vi "XCP and CCP - Curve Table Control.vi"() -> ()   [LabVIEW 2011]
doc: "Sample numeric display item."
uses:
  <vilib>/NI Veristand/Display Template Support/Display Template Support.llb/cluster_Screen Item Settings.ctl
  <vilib>/NI Veristand/Display Template Support/Display Template Support.llb/cluster_Graph Scale Settings.ctl
  <vilib>/NI Veristand/Display Template Support/Display Template Support.llb/cluster_Graph Plot Settings.ctl
  NationalInstruments.VeriStand.SystemStorage
  Tables/XCPCCP TBL1D.xctl
  Controls/Control Links.ctl
  Controls/ECUMC Item.ctl
  <vilib>/NI Veristand/Display Template Support/Display Template Support.llb/enum_Display Template Handler Minimal To Widget Msg.ctl
  <vilib>/NI Veristand/Display Template Support/Display Template Support.llb/enum_Display Template Handler Minimal To Workspace.ctl
  Controls/All Link Data.ctl
  Controls/LinkData.ctl
  <vilib>/ECUMC/NIVS/Support Files.llb/Item Properties.ctl
  <vilib>/ECUMC/NIVS/Support Files.llb/Address Property.ctl
  <vilib>/ECUMC/NIVS/Support Files.llb/Extension Property.ctl
  <vilib>/ECUMC/NIVS/Support Files.llb/Data Type Property.ctl
  <vilib>/ECUMC/NIVS/Support Files.llb/Byte Order Property.ctl
  <vilib>/ECUMC/NIVS/Support Files.llb/Maximum Property.ctl
  <vilib>/ECUMC/NIVS/Support Files.llb/Minimum Property.ctl
  <vilib>/ECUMC/NIVS/Support Files.llb/Read Only Property.ctl
  <vilib>/ECUMC/NIVS/Support Files.llb/Unit Property.ctl
  <vilib>/ECUMC/NIVS/Support Files.llb/Comment Property.ctl
  <vilib>/ECUMC/NIVS/Support Files.llb/X Dimension Property.ctl
  <vilib>/ECUMC/NIVS/Support Files.llb/Y Dimension Property.ctl
  <vilib>/ECUMC/NIVS/Support Files.llb/Is Virtual Property.ctl
  Tables/Limits TBL1D.ctl
  <vilib>/ECUMC/NIVS/Support Files.llb/Item Type.ctl
  SubVIs/Get Conn Status Chan Path.vi
  SubVIs/Check Link for Char or Meas.vi
  <vilib>/NI Veristand/Display Template Support/Display Template Support.llb/sub_Display Template Handler Custom.vi
  <vilib>/ECUMC/NIVS/Set Char Data.vi
  <vilib>/ECUMC/NIVS/Support Files.llb/Set Char Data (1d, TCP).vi
  <vilib>/NI Veristand/Execution/Workspace/NI VeriStand - Set Channel Value.vi
  <vilib>/NI Veristand/Execution/Workspace/NI VeriStand - Set Multiple Channel Values.vi
  <vilib>/NI Veristand/Execution/Workspace/NI VeriStand - Get Channel Value.vi
  <vilib>/NI Veristand/Execution/Workspace/NI VeriStand - Get Multiple Channel Values.vi
  <vilib>/NI Veristand/Execution/Workspace/NI VeriStand - Get System State.vi
  <vilib>/ECUMC/NIVS/Support Files.llb/Get Single Char Properties (TCP).vi
  <vilib>/ECUMC/NIVS/Get Char Data.vi
  <vilib>/ECUMC/NIVS/Support Files.llb/Get Single Char Data (TCP).vi
  <vilib>/ECUMC/NIVS/Get Meas Data.vi
  <vilib>/ECUMC/NIVS/Support Files.llb/Get Single Meas Data (TCP).vi
  <vilib>/NI Veristand/Execution/Workspace/NI VeriStand - Get Single Channel Value.vi
  <vilib>/NI Veristand/Execution/Workspace/NI_VS Workspace ExecutionAPI.lvlib
  <vilib>/ECUMC/NIVS/XCPCCP Add-On Execution API.lvlib
  <vilib>/ECUMC/NIVS/Support Files.llb/XCP and CCP Master Custom Device.lvlib
panel:
  in  "Links":T1
  out "Selected Parameter":string
  in  "TBL1D":cluster{"X":sgl[], "Y":sgl[]}(xcontrol)
  in  "NIVS.System Definition Root":refnum<k24>
  in  "Item.Data":T3
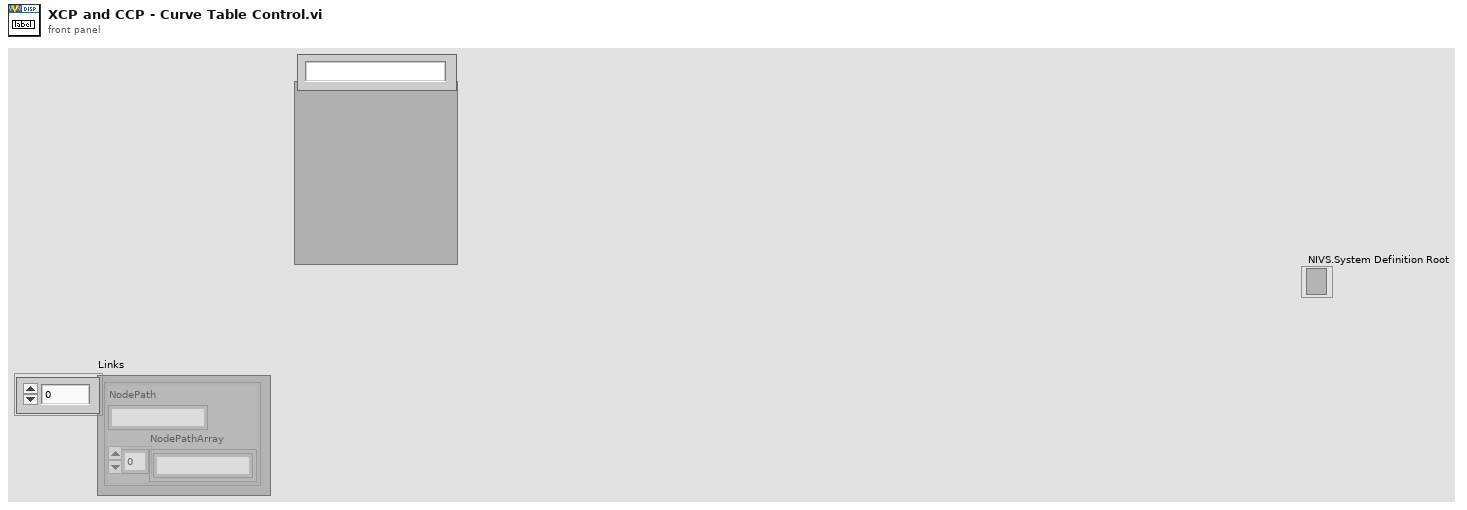
[diagram p1: front panel]
types:
  T1 = typedef "Control Links.ctl" = T2[]
  T2 = typedef "ECUMC Item.ctl" = cluster{"NodePath":string, "NodePathArray":string[]}
  T3 = typedef "cluster_Screen Item Settings.ctl" = cluster{"Template VI":string, "Position X":i32, "Position Y":i32, "Custom":string, "Show Title Bar":bool, "ID":i32, "Always On Top":bool, "Allow Resize":bool, "Allow Minimize":bool, "Allow Close":bool, "Size to Screen":bool, "Screen.ID":i32, "State":enum16{"Normal", "New"}, "Title":string, "Window Bounds":cluster{"[0]":i16, "[1]":i16, "[2]":i16, "[3]":i16}, "Channel Ref":u64, "Unit":string, "Default Units?":bool, "Flash Limit?":bool, "Color 1":u32, "Color 2":u32, "Color 3":u32, "Color 4":u32, "Bck Color":u32, "Fore Color":u32, "Limit 1":dbl, "Limit 2":dbl, "Limit 3":dbl, "Limit 4":dbl, "Limit Mode 1":i32, "Limit Mode 2":i32, "Limit Mode 3":i32, "Limit Mode 4":i32, "Scale Precision":i32, "Scale Min":dbl, "Scale Max":dbl, "Format":i32, "Precision":i32, "Background Type":i32, "IDs":i32[], "Units":string[], "Labels":string[], "Scale Factor":dbl, "Scale Offset":dbl, "YScale Index":u32[], "XScale":T4, "YScales":T4[], "Plots":T5[], "Update Period":dbl, "History Length":dbl, "My.Ref":refnum<vi>, "Is Control?":bool, "Channel Paths":string[], "Custom Data":variant}
  T4 = typedef "cluster_Graph Scale Settings.ctl" = cluster{"Format":u8, "Precision":u8, "Fit":u8, "Label":string, "Use Default Label":bool, "Label Visible":bool, "Min":dbl, "Max":dbl}
  T5 = typedef "cluster_Graph Plot Settings.ctl" = cluster{"Bar Style":u8, "Fill To":i16, "Fill/PtColor":u32, "Line Style":u8, "Line Width":u8, "Color":u32, "Interp":u8, "Point Style":u8}
  T6 = typedef "XCPCCP TBL1D.xctl/Limits TBL1D.ctl" = cluster{"Min X":sgl, "Max X":sgl, "MaxDiff X":sgl, "MaxGrad X":sgl, "Min Y":sgl, "Max Y":sgl, "MaxDiff Y":sgl}
  T7 = typedef "XCP and CCP Master Custom Device.lvlib/Item Properties.ctl" = cluster{"Common":cluster{"Address":T8, "Extension":T9, "Data Type":T10, "Byte Order":T11, "Maximum":T12, "Minimum":T13, "Read Only?":T14, "Unit":T15, "Comment":T16}, "Char Specific":cluster{"X Dimension":T17, "Y Dimension":T18, "char x axis":dbl[], "char y axis":dbl[], "char sizes":u32[]}, "Meas Specific":cluster{"Virtual?":T19}}
  T8 = typedef "XCP and CCP Master Custom Device.lvlib/Address Property.ctl" = u32
  T9 = typedef "XCP and CCP Master Custom Device.lvlib/Extension Property.ctl" = u8
  T10 = typedef "XCP and CCP Master Custom Device.lvlib/Data Type Property.ctl" = enum16{"UBYTE", "SBYTE", "UWORD", "SWORD", "ULONG", "SLONG", "FLOAT32_IEEE", "FLOAT64_IEEE"}
  T11 = typedef "XCP and CCP Master Custom Device.lvlib/Byte Order Property.ctl" = enum16{"Intel", "Motorola"}
  T12 = typedef "XCP and CCP Master Custom Device.lvlib/Maximum Property.ctl" = dbl
  T13 = typedef "XCP and CCP Master Custom Device.lvlib/Minimum Property.ctl" = dbl
  T14 = typedef "XCP and CCP Master Custom Device.lvlib/Read Only Property.ctl" = bool
  T15 = typedef "XCP and CCP Master Custom Device.lvlib/Unit Property.ctl" = string
  T16 = typedef "XCP and CCP Master Custom Device.lvlib/Comment Property.ctl" = string
  T17 = typedef "XCP and CCP Master Custom Device.lvlib/X Dimension Property.ctl" = u32
  T18 = typedef "XCP and CCP Master Custom Device.lvlib/Y Dimension Property.ctl" = u32
  T19 = typedef "XCP and CCP Master Custom Device.lvlib/Is Virtual Property.ctl" = bool
  T20 = typedef "All Link Data.ctl" = T21[]
  T21 = typedef "LinkData.ctl" = cluster{"Chns":string[], "InSys?":bool, "IP":string, "Port":u16}
  T22 = typedef "enum_Display Template Handler Minimal To Workspace.ctl" = cluster{"Operation":enum16{"SetCustomData", "DeleteItem"}, "Data":variant}
  T23 = typedef "enum_Display Template Handler Minimal To Widget Msg.ctl" = enum16{"Stop", "LaunchConfigDialog"}
  T24 = typedef "NI_VS Workspace ExecutionAPI.lvlib/WorkspaceAPI.ctl" = refnum<k24>
  T25 = typedef "NI_VS Workspace ExecutionAPI.lvlib/SystemStateEventRef.ctl" = cluster{"CustDatRef":refnum<user-event>, "EvtRef":refnum<k27>}
  T26 = typedef "NI_VS Workspace ExecutionAPI.lvlib/SystemStateRegEventRef.ctl" = refnum<event-registration>
  T27 = cluster{"Event Registration Refnum":refnum<event-registration>, "SystemChangeEventRef":T26}
  T28 = typedef "XCP and CCP Master Custom Device.lvlib/Item Type.ctl" = enum16{"Scalar Characteristic", "Curve Characteristic", "Field Characteristic", "Measurement"}
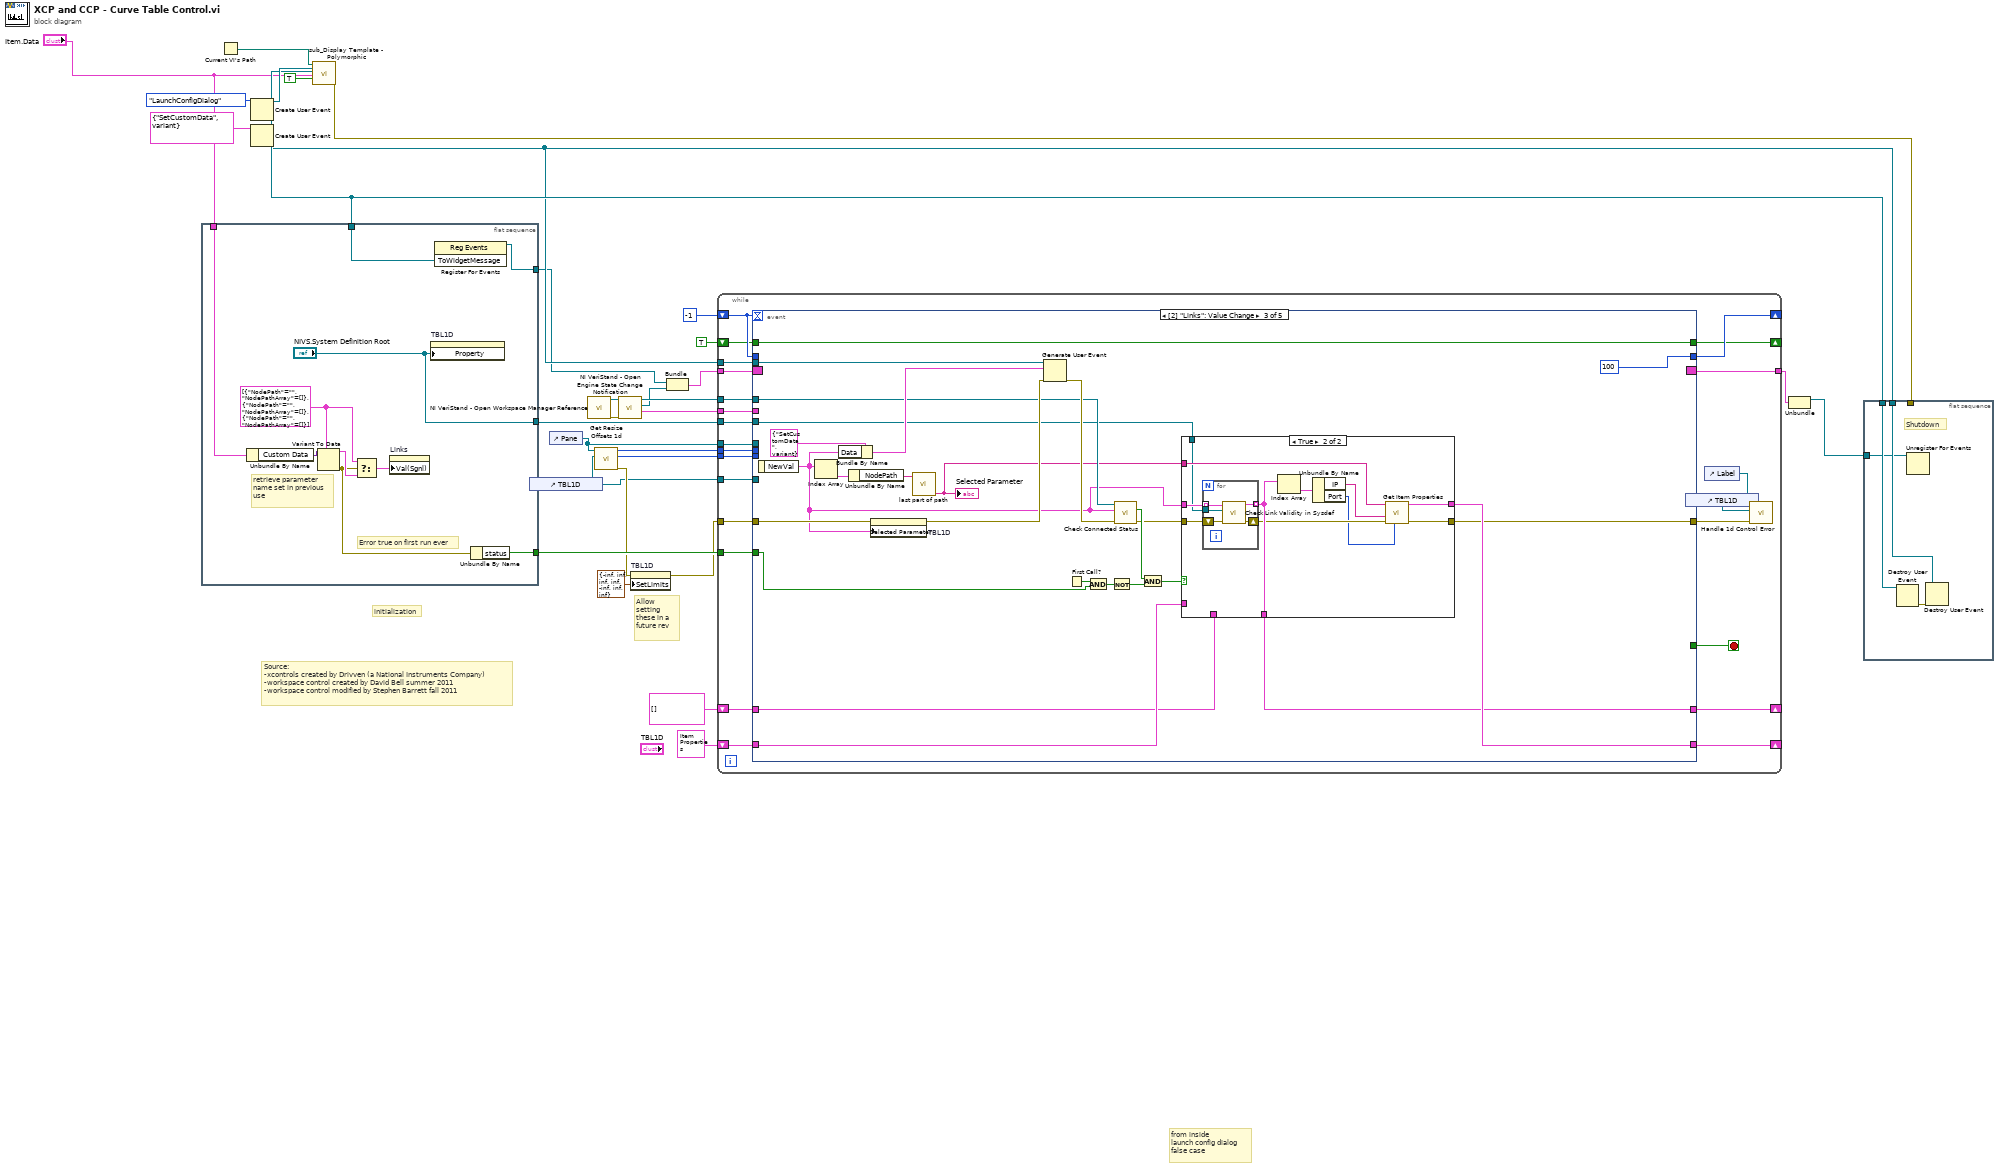
[diagram p0: block diagram]
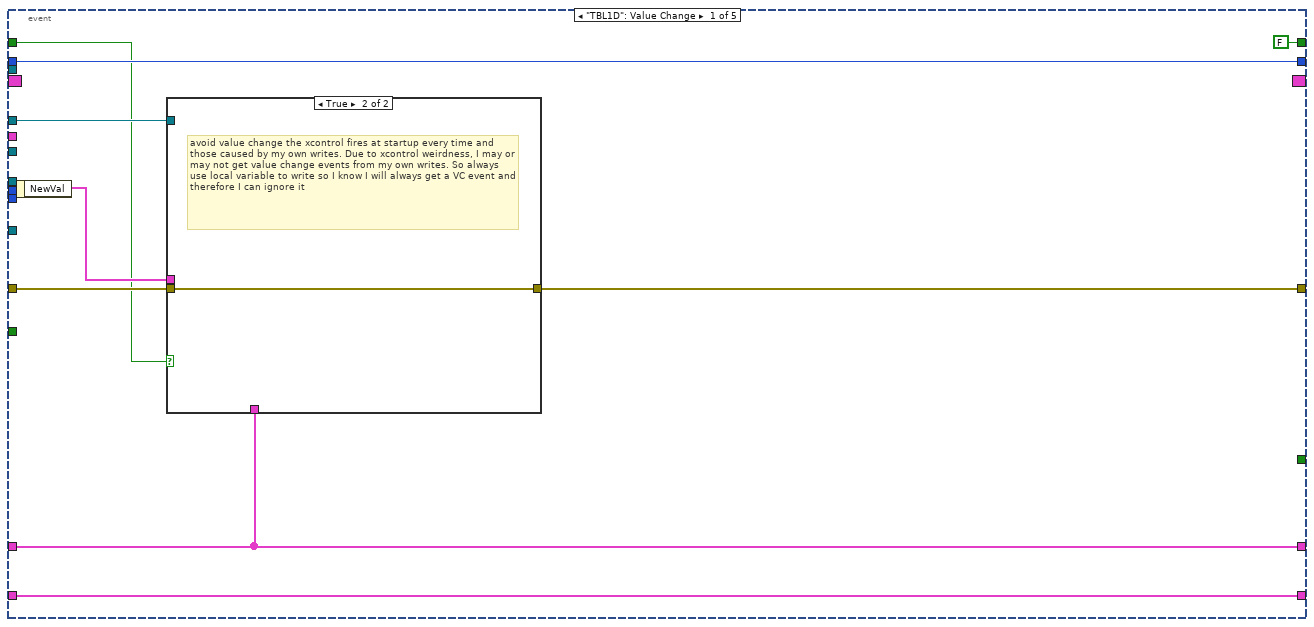
[diagram p2: hidden frame]
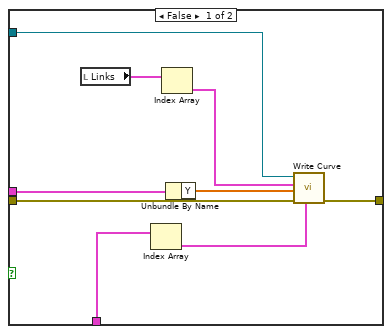
[diagram p3: hidden frame]
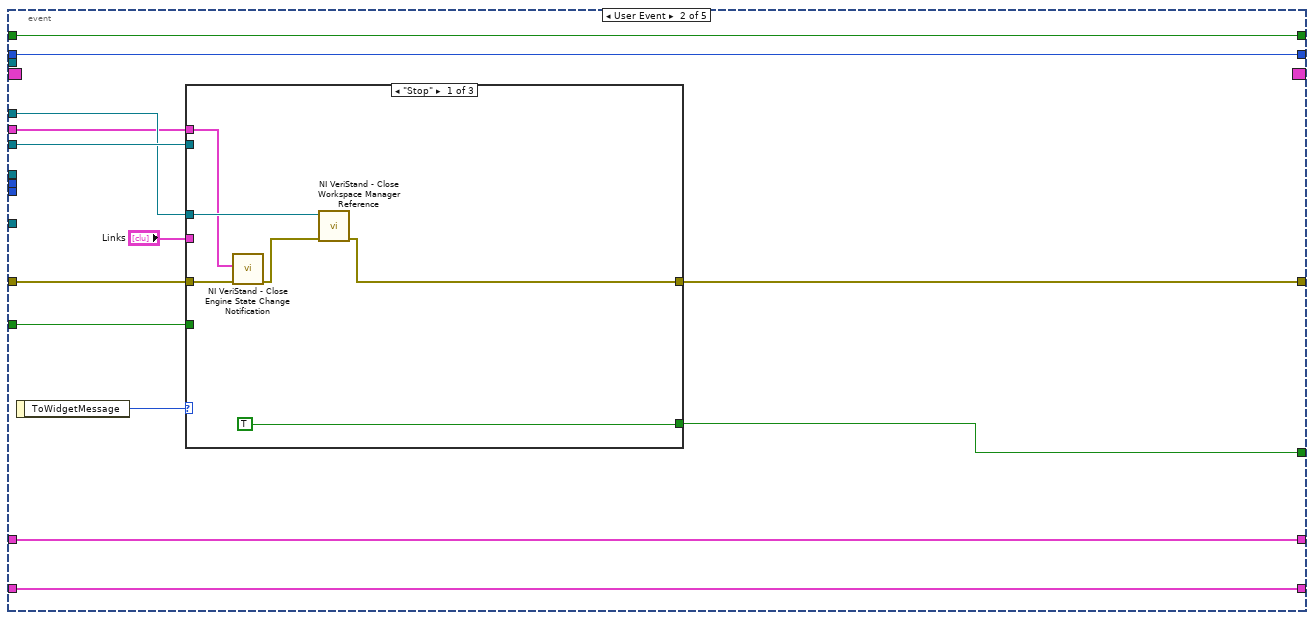
[diagram p4: hidden frame]
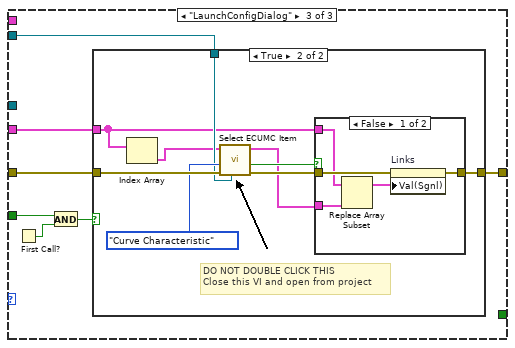
[diagram p6: hidden frame]
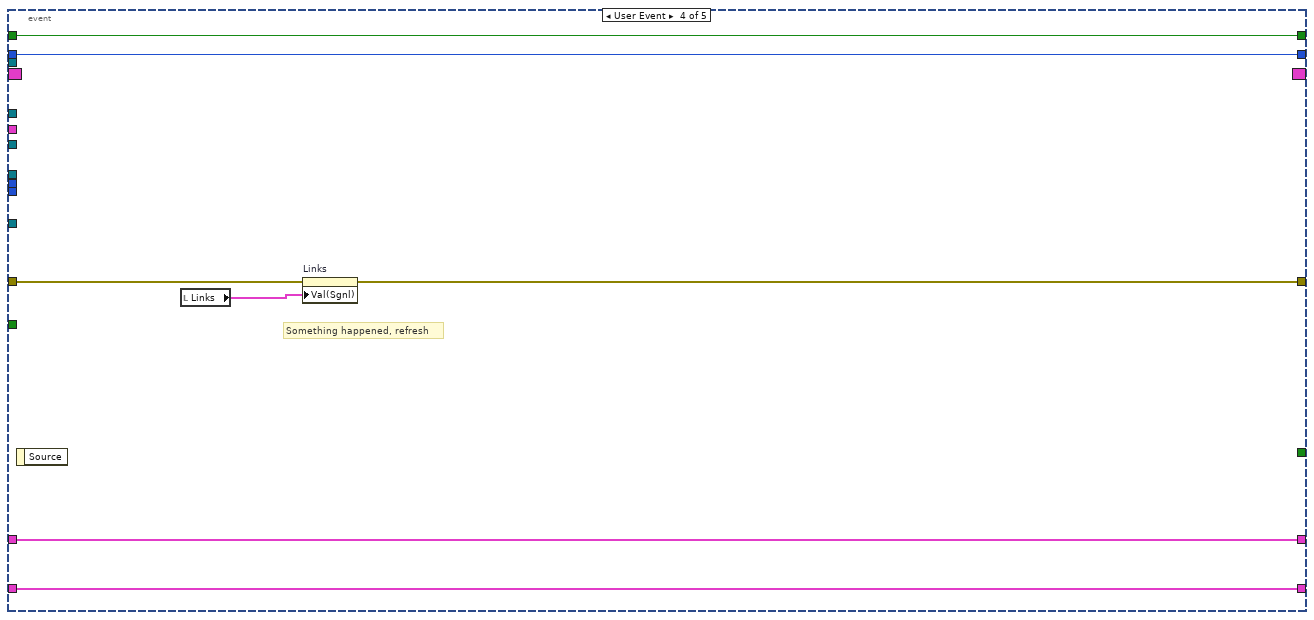
[diagram p10: hidden frame]
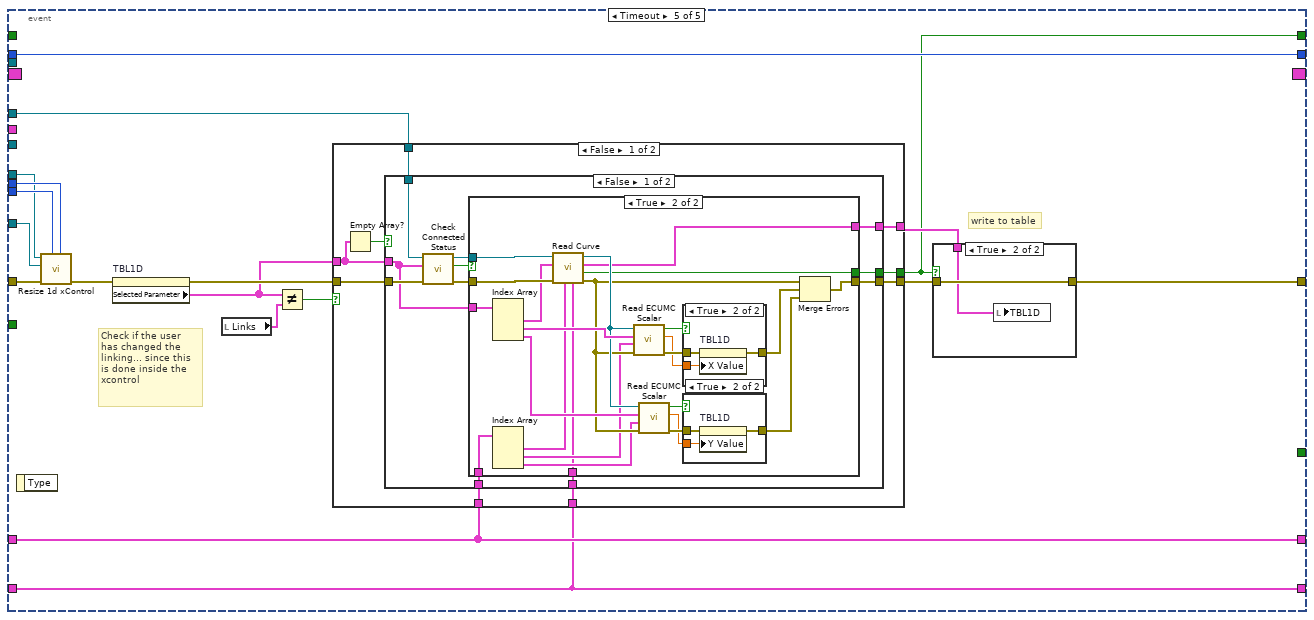
[diagram p11: hidden frame]
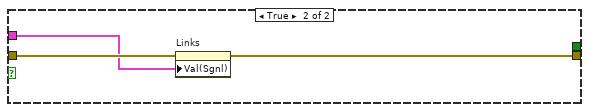
[diagram p17: hidden frame]
diagram:
  # "Source: \n-xcontrols created by Drivven (a National Instruments Company)\n-workspace control created by David Bell summer 2011\n-workspace control modified by Stephen Barrett fall 2011"
  # "Allow setting these in a future rev"
  # "initialization"
  # "from inside\nlaunch config dialog\nfalse case"
  n1 = flat-sequence {
    tunnel: [w40] -> w11
    tunnel: w28 -> [w39]
    tunnel: "Item.Data" -> [w37]
    tunnel: ["NIVS.System Definition Root"] -> w22
    tunnel: [w32] -> w21
    frame #0 {
      w31 = T1 [{"NodePath"="", "NodePathArray"=[]}, {"NodePath"="", "NodePathArray"=[]}, {"NodePath"="", "NodePathArray"=[]}] ("Links")
      # "Error true on first run ever"
      # "retrieve parameter\nname set in previous\nuse"
      n2 = Unbundle By Name(w37) -> ("Custom Data"=w38:variant)
      n3 = Variant To Data(type=w31, Variant=w38) -> (data=w34:T1, error out=w33:errorcluster)  [unwired: 1 in]
      n4 = Select(t=w31, s=w33, f=w34) -> (s? t:f=w35:T1)
      n5 = property on="Links" class="Arr (strict)"("Val(Sgnl)"=w35) -> ()  [unwired: 2 in, 2 out]
      n6 = property on="TBL1D" class="XCPCCP TBL1D (strict)"("Property"="NIVS.System Definition Root") -> ()  [unwired: 2 in, 2 out]
      n7 = register-events(w39) -> (reference out=w40:refnum<event-registration>)  [unwired: 2 in, 1 out]
      n8 = Unbundle By Name(w33) -> ("status"=w32:bool)
    }
  }
  n9 = Current VI's Path() -> (path=w26:path)
  n10 = Create User Event(user event datatype=enum_Display_Template_Handler_Minimal_To_Widget_Msg."LaunchConfigDialog" ("ToWidgetMessage")) -> (user event=w28:refnum<user-event>)  [unwired: 1 in, 1 out]
  n11 = Create User Event(user event datatype=T22 {"Operation"=enum."SetCustomData", "Data"=variant} ("Data")) -> (user event=w25:refnum<user-event>)  [unwired: 1 in, 1 out]
  n12 = call-poly <vilib>:"sub_Display Template - Polymorphic.vi"("Parent.Path"=w26, "ToWidgetEvent"=w28, "ToWorkspace"=w25, "Item.Data"="Item.Data", "Resizable"=TRUE) -> ("error out"=w30:errorcluster)  [unwired: 1 in, 13 out]
  n13 = control-ref of="TBL1D"() -> (w5:refnum<vi>)
  n14 = control-ref of="Pane"() -> (w16:refnum<vi>)
  n15 = call <vilib>:"NI VeriStand - Open Workspace Manager Reference.vi"() -> ("error out"=w13:errorcluster, "WorkspaceManager"=w12:T24)  [unwired: 10 in]
  n16 = call "Get Resize Offsets 1d.vi"("TBL1D Refnum"=w5, "Pane in"=w16) -> ("error out"=w19:errorcluster, "Width Offset"=w17:u32, "Height Offset"=w18:u32)  [unwired: 7 in]
  n17 = call <vilib>:"NI VeriStand - Open Engine State Change Notification.vi"("error in (no error)"=w13, "WorkspaceManager in"=w12) -> ("SystemStateRefs"=w7:T25, "SystemChangeEventRef"=w9:T26, "WorkspaceManager out"=w10:T24)  [unwired: 6 in, 1 out]
  n18 = property on="TBL1D" class="XCPCCP TBL1D (strict)"(error in=w19, "SetLimits"=T6 {"Min X"=-inf, "Max X"=inf, "MaxDiff X"=inf, "MaxGrad X"=inf, "Min Y"=-inf, "Max Y"=inf, "MaxDiff Y"=inf}) -> (error out=w20:errorcluster)  [unwired: 1 in, 1 out]
  n19 = Bundle("Event Registration Refnum"=w11, "SystemChangeEventRef"=w9) -> (w8:T27)  [unwired: 1 in]
  n20 = while {
    tunnel: w8 -> [w64]
    tunnel: [w63] -> w6
    tunnel: w25 -> [w62]
    tunnel: w20 -> [w60]
    tunnel: w10 -> [w61]
    tunnel: w22 -> [w59]
    tunnel: w21 -> [w58]
    tunnel: w18 -> [w57]
    tunnel: w17 -> [w56]
    tunnel: w16 -> [w55]
    tunnel: w5 -> [w54]
    shift-right: [w48] -> _
    shift-left: T20 [] ("All LinkData") -> [w46]
    shift-right: [w49] -> _
    shift-left: T7 {"Common"={"Address"=0, "Extension"=0, "Data Type"=enum."UBYTE", "Byte Order"=enum."Intel", "Maximum"=0.0, "Minimum"=0.0, "Read Only?"=FALSE, "Unit"="", "Comment"=""}, "Char Specific"={"X Dimension"=0, "Y Dimension"=0, "char x axis"=[], "char y axis"=[], "char sizes"=[]}, "Meas Specific"={"Virtual?"=FALSE}} ("Properties") -> [w47]
    tunnel: w7 -> [w45]
    shift-right: [w44] -> _
    shift-left: -1 -> [w43]
    shift-right: [w42] -> _
    shift-left: TRUE -> [w41]
    stop <- w53 stop-if-true
    n21 = event shown="[2] \"Links\": Value Change" {
      selector: w64 -> [_ _ _ _ _]
      dyn-events: [_ _ _ _ _] -> w63
      timeout: w43 -> [_ _ _ _ _]
      tunnel: w62 -> [_ _ w150 _ _]
      tunnel: [_ w96 _ _ _] -> w53
      tunnel: w61 -> [w72 w93 w144 _ w186]
      tunnel: w60 -> [w73 w92 w149 w178 w195]
      tunnel: w59 -> [_ w94 w134 _ _]
      tunnel: w58 -> [_ w91 w140 _ _]
      tunnel: w57 -> [_ _ _ _ w192]
      tunnel: w56 -> [_ _ _ _ w193]
      tunnel: w55 -> [_ _ _ _ w191]
      tunnel: w54 -> [_ _ _ _ w190]
      tunnel: [w71 w88 w129 w176 w181] -> w52
      tunnel: [w68 w86 w133 w174 w184] -> w49
      tunnel: [w69 w87 w132 w175 w185] -> w48
      tunnel: w47 -> [w68 w86 w131 w174 w184]
      tunnel: w46 -> [w69 w87 w130 w175 w185]
      tunnel: w45 -> [_ w89 _ _ _]
      tunnel: [w67 w85 100 w173 w180] -> w44
      tunnel: w43 -> [w67 w85 _ w173 w180]
      tunnel: [FALSE ("NewValue") w84 w127 w172 w179] -> w42
      tunnel: w41 -> [w66 w84 w127 w172 _]
      event "TBL1D": Value Change {
        n22 = event-data() -> ("NewVal"=w70:cluster{"X":sgl[], "Y":sgl[]})  [unwired: 1 in]
        n23 = case shown="True" w66 {
          tunnel: w73 -> [w82 w83]
          tunnel: w72 -> [w81 _]
          tunnel: [w80 w83] -> w71
          tunnel: w70 -> [w79 _]
          tunnel: w69 -> [w78 _]
          frame False {
            n24 = local read "Links"() -> (w77:T1)
            n25 = Index Array(array=w78) -> (element=w75:T21)  [unwired: 1 in]
            n26 = Index Array(array=w77) -> (element=w76:T2)  [unwired: 1 in]
            n27 = Unbundle By Name(w79) -> ("Y"=w74:sgl[])
            n28 = call "Write Curve.vi"("LinkData"=w75, "Error In"=w82, "Characteristic Curve Values"=w74, "Link"=w76, "WorkspaceManager"=w81) -> ("Error Out"=w80:errorcluster)  [unwired: 5 in, 1 out]
          }
          frame True {
            # "avoid value change the xcontrol fires at startup every time and those caused by my own writes. Due to xcontrol weirdness, I may or may not get value change events from my own writes. So always use local variable to write so I know I will always get a VC event and therefore I can ignore it"
          }
        }
      }
      event User Event {
        n29 = event-data() -> ("ToWidgetMessage"=w95:T23)  [unwired: 1 in]
        n30 = case shown="\"Stop\"" w95 {
          tunnel: [TRUE ("1-D array?") _ _] -> w96
          tunnel: w94 -> [_ _ w110]
          tunnel: w93 -> [w101 _ _]
          tunnel: "Links" -> [_ _ w107]
          tunnel: w92 -> [w99 w103 w109]
          tunnel: [w100 w103 w108] -> w88
          tunnel: w91 -> [_ _ w106]
          tunnel: w89 -> [w97 _ _]
          frame "Stop" {
            n31 = call <vilib>:"NI VeriStand - Close Engine State Change Notification.vi"("error in (no error)"=w99, "SystemStateRefs"=w97) -> ("error out"=w98:errorcluster)  [unwired: 9 in]
            n32 = call <vilib>:"NI VeriStand - Close Workspace Manager Reference.vi"("error in (no error)"=w98, "WorkspaceManager"=w101) -> ("error out"=w100:errorcluster)  [unwired: 9 in]
          }
          frame Default {
          }
          frame "LaunchConfigDialog" {
            n33 = First Call?() -> (First Call?: T/F=w104:bool)
            n34 = And(x=w106, y=w104) -> (x .and. y?=w105:bool)
            n35 = case shown="True" w105 {
              tunnel: w110 -> [_ w116]
              tunnel: w107 -> [_ w115]
              tunnel: w109 -> [w111 w119]
              tunnel: [w111 w120] -> w108
              frame False {
              }
              frame True {
                # "DO NOT DOUBLE CLICK THIS\nClose this VI and open from project"
                n36 = Index Array(array=w115) -> (element=w114:T2)  [unwired: 1 in]
                n37 = call "Select ECUMC Item.vi"("NIVS.System Definition Root"=w116, "error in (no error)"=w119, "Item Type"=Item_Type."Curve Characteristic", "Link In"=w114) -> ("error out"=w118:errorcluster, "Canceled?"=w113:bool, "Link Out"=w112:T2)  [unwired: 5 in]
                n38 = case shown="False" w113 {
                  tunnel: w118 -> [w125 w126]
                  tunnel: [w123 w126] -> w120
                  tunnel: w115 -> [w122 _]
                  tunnel: w112 -> [w121 _]
                  frame False {
                    n39 = Replace Array Subset(array=w122, new element=w121) -> (w124:T1)  [unwired: 1 in]
                    n40 = property on="Links" class="Arr (strict)"(error in=w125, "Val(Sgnl)"=w124) -> (error out=w123:errorcluster)  [unwired: 1 in, 1 out]
                  }
                  frame True {
                  }
                }
              }
            }
          }
        }
      }
      event Value Change {
        n41 = event-data() -> ("NewVal"=w136:T1)  [unwired: 1 in]
        n42 = Index Array(array=w136) -> (element=w147:T2)  [unwired: 1 in]
        n43 = Bundle By Name(cluster=T22 {"Operation"=enum."SetCustomData", "Data"=variant} ("event data"), "Data"=w136) -> (w152:T22)
        n44 = Unbundle By Name(w147) -> ("NodePath"=w146:string)
        n45 = property on="TBL1D" class="XCPCCP TBL1D (strict)"(error in=w149, "Selected Parameter"=w136) -> (error out=w148:errorcluster)  [unwired: 1 in, 1 out]
        n46 = call "last part of path.vi"("String"=w146) -> ("Last Part"=w135:string)  [unwired: 10 in]
        "Selected Parameter" <- w135
        n47 = Generate User Event(user event=w150, event data cluster=w152, error in=w148) -> (error out=w145:errorcluster)  [unwired: 1 out]
        n48 = First Call?() -> (First Call?: T/F=w141:bool)
        n49 = And(x=w141, y=w140) -> (x .and. y?=w142:bool)
        n50 = Not(x=w142) -> (.not. x?=w143:bool)
        n51 = call "Check Connected Status.vi"("Error In"=w145, "Links"=w136, "WorkspaceManager in"=w144) -> ("Error Out"=w138:errorcluster, "Connected?"=w139:bool)  [unwired: 6 in, 1 out]
        n52 = And(x=w139, y=w143) -> (x .and. y?=w137:bool)
        n53 = case shown="True" w137 {
          tunnel: w138 -> [w155 w166]
          tunnel: w136 -> [_ w165]
          tunnel: [w153 w164] -> w132
          tunnel: w135 -> [_ w162]
          tunnel: [w155 w159] -> w129
          tunnel: [w154 w158] -> w133
          tunnel: w131 -> [w154 _]
          tunnel: w130 -> [w153 _]
          tunnel: w134 -> [_ w156]
          frame False {
          }
          frame True {
            n54 = for {
              shift-right: [w170] -> w163
              shift-left: w166 -> [w171]
              tunnel: w165 -> [w169] mode=indexing
              tunnel: w156 -> [w167]
              tunnel: [w168] -> w164 mode=indexing
              n55 = call "Check Link Validity in Sysdef.vi"("error in (no error)"=w171, "SysDef Root"=w167, "Link"=w169) -> ("error out"=w170:errorcluster, "LinkData"=w168:T21)  [unwired: 7 in]
            }
            n56 = Index Array(array=w164) -> (element=w157:T21)  [unwired: 1 in]
            n57 = Unbundle By Name(w157) -> ("IP"=w161:string, "Port"=w160:u16)
            n58 = call-poly <vilib>:"Get Item Properties.vi"("Port"=w160, "error in (no error)"=w163, "IP or DNS Name"=w161, "Characteristic"=w162) -> ("error out"=w159:errorcluster, "Properties"=w158:T7)  [unwired: 6 in]
          }
        }
      }
      event User Event {
        # "Something happened, refresh"
        n59 = event-data() -> ()  [unwired: 1 in, 1 out]
        n60 = local read "Links"() -> (w177:T1)
        n61 = property on="Links" class="Arr (strict)"(error in=w178, "Val(Sgnl)"=w177) -> (error out=w176:errorcluster)  [unwired: 1 in, 1 out]
      }
      event Timeout {
        # "Check if the user has changed the linking... since this is done inside the xcontrol"
        # "write to table"
        n62 = event-data() -> ()  [unwired: 1 in, 1 out]
        n63 = call "Resize 1d xControl.vi"("Height Offset"=w192, "Width Offset"=w193, "error in (no error)"=w195, "Control in"=w190, "Pane"=w191) -> ("error out"=w194:errorcluster)  [unwired: 6 in]
        n64 = property on="TBL1D" class="XCPCCP TBL1D (strict)"(error in=w194) -> (error out=w188:errorcluster, "Selected Parameter"=w187:T1)  [unwired: 1 in, 1 out]
        n65 = local read "Links"() -> (w196:T1)
        n66 = Not Equal?(x=w187, y=w196) -> (x != y?=w189:bool)
        n67 = case shown="False" w189 {
          tunnel: w188 -> [w208 w256]
          tunnel: w187 -> [w207 w255]
          tunnel: w186 -> [w205 _]
          tunnel: [w204 w254] -> w183
          tunnel: [w203 _] -> w182
          tunnel: w185 -> [w202 _]
          tunnel: w184 -> [w201 _]
          tunnel: [w200 _] -> w179
          frame False {
            n68 = Empty Array?(array=w207) -> (empty?=w206:bool)
            n69 = case shown="False" w206 {
              tunnel: w208 -> [w219 w253]
              tunnel: w207 -> [w214 _]
              tunnel: w205 -> [w218 _]
              tunnel: [w213 w253] -> w204
              tunnel: [w212 _] -> w203
              tunnel: w202 -> [w211 _]
              tunnel: w201 -> [w210 _]
              tunnel: [w209 _] -> w200
              frame False {
                n70 = call "Check Connected Status.vi"("Error In"=w219, "Links"=w214, "WorkspaceManager in"=w218) -> ("Error Out"=w216:errorcluster, "Connected?"=w217:bool, "WorkspaceManager out"=w215:T24)  [unwired: 6 in]
                n71 = case shown="True" w217 {
                  tunnel: w216 -> [w220 w244]
                  tunnel: w215 -> [_ w241]
                  tunnel: w214 -> [_ w243]
                  tunnel: [w220 w228] -> w213
                  tunnel: [_ w227] -> w212
                  tunnel: w211 -> [_ w223]
                  tunnel: w210 -> [_ w222]
                  tunnel: [_ w221] -> w209
                  frame False {
                  }
                  frame True {
                    n72 = Index Array(array=w243) -> (element #1=w242:T2, element #2=w240:T2, element #3=w238:T2)  [unwired: 3 in]
                    n73 = Index Array(array=w223) -> (element #1=w226:T21, element #2=w225:T21, element #3=w224:T21)  [unwired: 3 in]
                    n74 = call "Read Curve.vi"("Properties"=w222, "LinkData"=w226, "Error In"=w244, "Link"=w242, "WorkspaceManager"=w241) -> ("Error Out"=w231:errorcluster, "NewValue"=w221:bool, "TBL1D"=w227:cluster{"X":sgl[], "Y":sgl[]}, "WorkspaceManager out"=w239:T24)  [unwired: 3 in]
                    n75 = call "Read ECUMC Scalar.vi"("Error In"=w231, "LinkData"=w225, "Link"=w240, "WorkspaceManager"=w239) -> ("Error Out"=w237:errorcluster, "Value"=w235:dbl, "Changed?"=w236:bool)  [unwired: 5 in]
                    n76 = call "Read ECUMC Scalar.vi"("Error In"=w231, "LinkData"=w224, "Link"=w238, "WorkspaceManager"=w239) -> ("Error Out"=w233:errorcluster, "Value"=w232:dbl, "Changed?"=w234:bool)  [unwired: 5 in]
                    n77 = case shown="True" w236 {
                      tunnel: w237 -> [w249 w252]
                      tunnel: [w249 w251] -> w230
                      tunnel: w235 -> [_ w250]
                      frame False {
                      }
                      frame True {
                        n78 = property on="TBL1D" class="XCPCCP TBL1D (strict)"(error in=w252, "X Value"=w250) -> (error out=w251:errorcluster)  [unwired: 1 in, 1 out]
                      }
                    }
                    n79 = case shown="True" w234 {
                      tunnel: w233 -> [w245 w248]
                      tunnel: [w245 w247] -> w229
                      tunnel: w232 -> [_ w246]
                      frame False {
                      }
                      frame True {
                        n80 = property on="TBL1D" class="XCPCCP TBL1D (strict)"(error in=w248, "Y Value"=w246) -> (error out=w247:errorcluster)  [unwired: 1 in, 1 out]
                      }
                    }
                    n81 = Merge Errors(w231, w230, w229) -> (w228:errorcluster)
                  }
                }
              }
              frame True {
              }
            }
          }
          frame True {
            n82 = property on="Links" class="Arr (strict)"(error in=w256, "Val(Sgnl)"=w255) -> (error out=w254:errorcluster)  [unwired: 1 in, 1 out]
          }
        }
        n83 = case shown="True" w179 {
          tunnel: w183 -> [w197 w199]
          tunnel: w182 -> [_ w198]
          tunnel: [w197 w199] -> w181
          frame False {
          }
          frame True {
            n84 = local write "TBL1D"(w198) -> ()
          }
        }
      }
    }
    n85 = control-ref of="TBL1D"() -> (w51:refnum<vi>)
    n86 = control-ref of="Label"() -> (w50:refnum<vi>)
    n87 = call "Handle 1d Control Error.vi"("Error In"=w52, "TBL1D Refnum"=w51, "Label"=w50) -> ()  [unwired: 9 in]
  }
  n88 = Unbundle(w6) -> ("Event Registration Refnum"=w3:refnum<event-registration>)  [unwired: 1 out]
  n89 = flat-sequence {
    tunnel: w30 -> [_]
    tunnel: w28 -> [w260]
    tunnel: w25 -> [w259]
    tunnel: w3 -> [w257]
    frame #0 {
      # "Shutdown"
      n90 = Destroy User Event(user event=w260) -> (error out=w258:errorcluster)  [unwired: 1 in]
      n91 = Unregister For Events(event registration refnum=w257) -> ()  [unwired: 1 in, 1 out]
      n92 = Destroy User Event(user event=w259, error in=w258) -> ()  [unwired: 1 out]
    }
  }
